vi "数值控件.vi"() -> ()   [LabVIEW 2014]
panel:
  in  "数值DBL":dbl=1000.0 caption="数值"
  in  "10进制":dbl=1000.0 caption="数值"
  in  "SI符号显示":dbl=1000.0 caption="数值" format="%#_p"
  in  "2进制":i32=10 caption="数值" format="%.0b"
  in  "8进制":i32=10 caption="数值" format="%.0o"
  in  "16进制":i32=10 caption="数值" format="%.0x"
  in  "数值":i32
  # "数值控件的组成和进制转换"
  # "标签"
  # "增量、减量按钮"
  # "数值输入和显示"
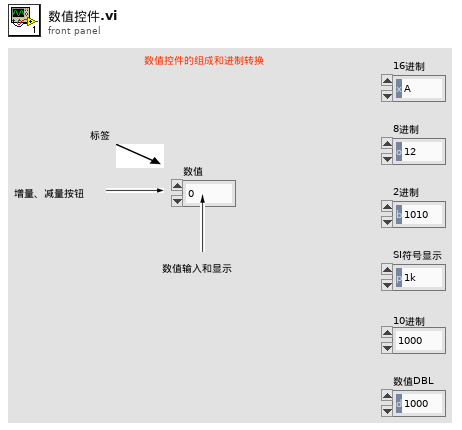
[diagram p1: front panel]
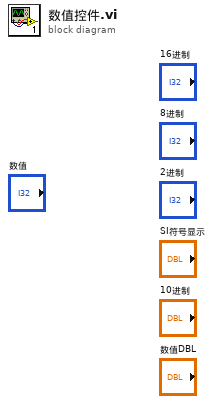
[diagram p0: block diagram]
diagram:
